vi "FGA Get Waypoint IDs.vi"() -> (0 "elements UID list":u16[](array[numeric]))   [LabVIEW 2009]
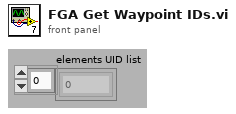
[diagram p1: front panel]
types:
  T1 = typedef "RequestIDRec.ctl" = cluster{"RequestId":u8, "Element List":T2[]}
  T2 = typedef "ElementRec.ctl" = cluster{"ElementUID":u16, " PreviousUID":u16, " NextUID":u16, "LocalWaypointRec":T3}
  T3 = typedef "LocalWaypointRec.ctl" = cluster{"Presence Vector":u8, " X":dbl, " Y":dbl, " Z":dbl, "Roll":dbl, "Pitch":dbl, "Yaw":dbl, "Waypoint Tolerance":dbl, "Path Tolerance":dbl, "Is Active?":bool}
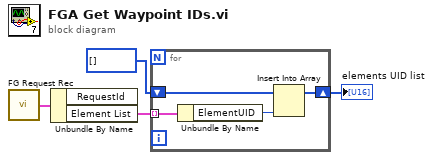
[diagram p0: block diagram]
diagram:
  n1 = call "FG Request Rec.vi"() -> ("Request out"=w2:T1)  [unwired: 2 in]
  n2 = Unbundle By Name(w2) -> ("Element List"=w1:T2[])  [unwired: 1 out]
  n3 = for {
    tunnel: w1 -> [w8] mode=indexing
    shift-right: [w6] -> w4
    shift-left: u16[] [] -> [w5]
    n4 = Unbundle By Name(w8) -> ("ElementUID"=w7:u16)
    n5 = Insert Into Array(array=w5, new element=w7) -> (w6:u16[])  [unwired: 1 in]
  }
  "elements UID list" <- w4
